vi "Load Plugins.vi"(8 "error in (no error)":errorcluster, 11 "Plugin Directories":path[](array[path])) -> (0 "error out":errorcluster, 3 "Plugin Array":T1[](array[typedef]))   [LabVIEW 2020, in "RxnRover.lvlib" / "Plugin Manager.lvlib"]
doc: "The core loader for plugins which initializes a Plugin Array, reads their configuration files and outputs a completed Plugin Array. This VI is currently called by Load Details and Filter Plugins. This VI calls several helper VIs starting with Read Plugins INI."
uses:
  Plugin Manager.lvlib
  Plugin Details.ctl
  Plugin Servers/Controller/Controller Type.ctl
  Plugin Types.ctl
  Config Error.ctl
  Plugin Servers/Controller/Generic Plugin.lvclass
  logging/logging.lvlib
panel:
  out "All Files in Dir":path[](array[path])
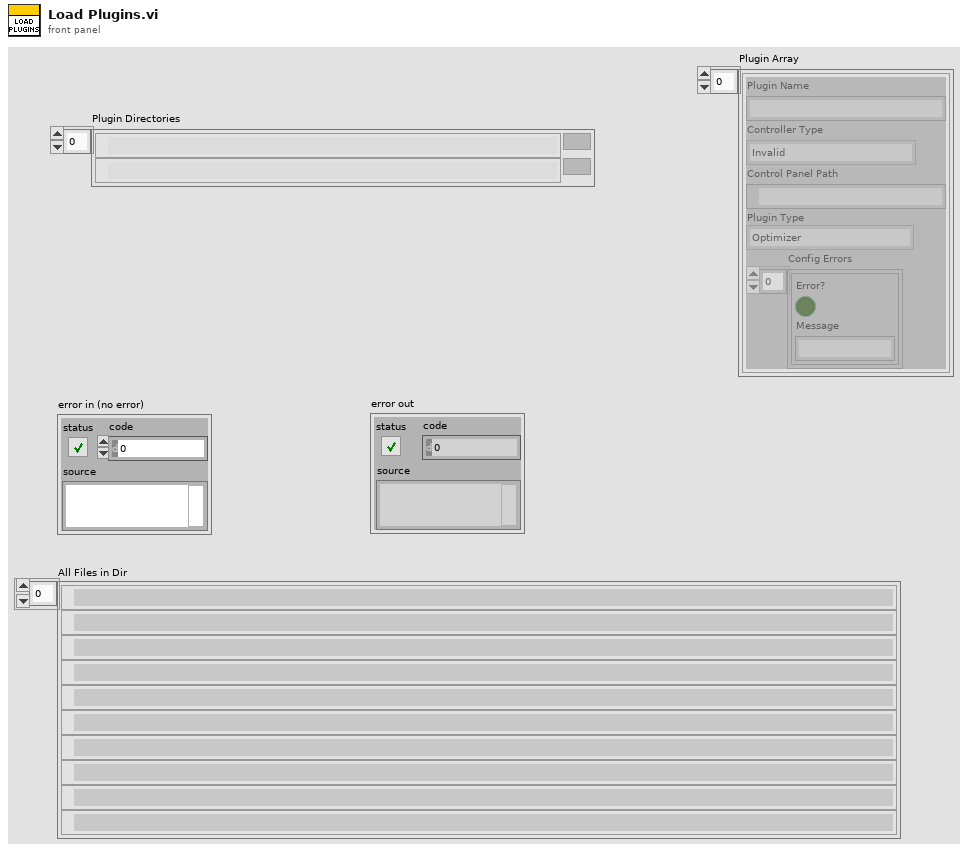
[diagram p1: front panel]
types:
  T1 = typedef "RxnRover.lvlib/Plugin Manager.lvlib/Plugin Details.ctl" = cluster{"Plugin Name":string, "Controller Type":T2, "Control Panel Path":path, "Plugin Type":T3, "Config Errors":T4[]}
  T2 = typedef "RxnRover.lvlib/Generic Plugin.lvclass/Controller Type.ctl" = enum16{"Invalid", "Temperature Controller", "Pump Controller", "Syringe Pump", "Generic Optimizer", "LC Parser", "Passive Hardware"}
  T3 = typedef "RxnRover.lvlib/Plugin Manager.lvlib/Plugin Types.ctl" = enum16{"Invalid", "Optimizer", "Analyzer", "Hardware"}
  T4 = typedef "RxnRover.lvlib/Plugin Manager.lvlib/Config Error.ctl" = cluster{"Error?":bool, "Message":string}
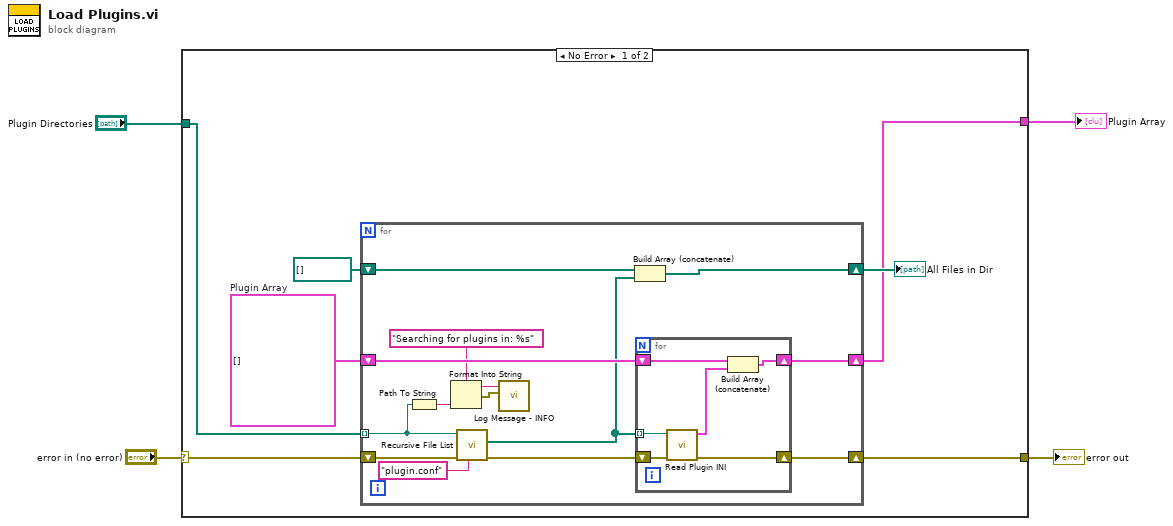
[diagram p0: block diagram]
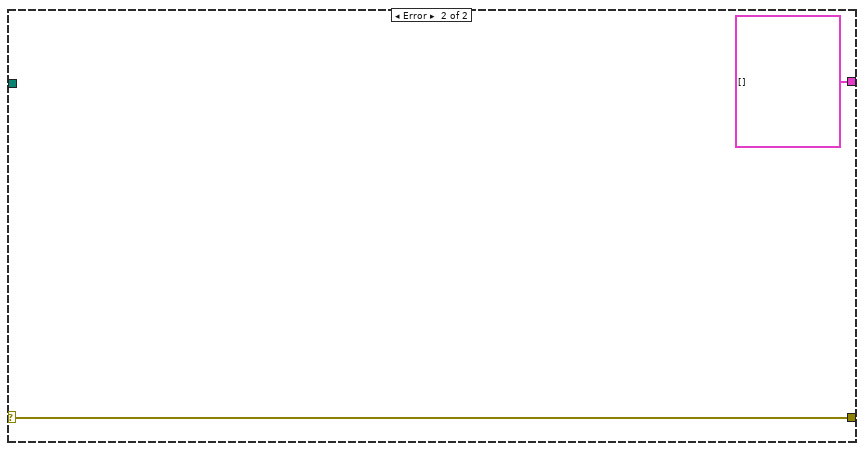
[diagram p2: hidden frame]
diagram:
  n1 = case shown="No Error" "error in (no error)" {
    selector: "error in (no error)" -> [w11 w33]
    tunnel: [w10 w33] -> w3
    tunnel: "Plugin Directories" -> [w8 _]
    tunnel: [w5 T1[] [] ("Plugin Array")] -> w2
    frame No Error {
      w9 = T1[] []  # Plugin Array
      n2 = for {
        shift-right: [w22] -> w10
        shift-left: w11 -> [w25]
        shift-right: [w20] -> w5
        shift-left: w9 -> [w21]
        tunnel: w8 -> [w13] mode=indexing
        shift-right: [w18] -> w6
        shift-left: path[] [] ("All Files in Dir") -> [w19]
        n3 = Path To String(path=w13) -> (string=w12:string)
        n4 = Format Into String(format string="Searching for plugins in: %s", w12) -> (resulting string=w15:string, error out=w16:errorcluster)  [unwired: 2 in]
        n5 = call <vilib>:"Recursive File List.vi"("pattern"="plugin.conf", "error in (no error)"=w25, "Folder Path"=w13) -> ("error out"=w23:errorcluster, "All Files in Dir"=w17:path[])  [unwired: 4 in, 3 out]
        n6 = call "Log Message - INFO.vi"("error in (no error)"=w16, "Message"=w15) -> ()  [unwired: 9 in, 1 out]
        n7 = Build Array (concatenate)(w19, w17) -> (w18:path[])
        n8 = for {
          shift-right: [w30] -> w22
          shift-left: w23 -> [w31]
          tunnel: w17 -> [w29] mode=indexing
          shift-right: [w27] -> w20
          shift-left: w21 -> [w28]
          n9 = call "Read Plugin INI.vi"("error in (no error)"=w31, "INI file"=w29) -> ("error out"=w30:errorcluster, "Plugin Details"=w26:T1)  [unwired: 8 in]
          n10 = Build Array (concatenate)(w28, w26) -> (w27:T1[])
        }
      }
      "All Files in Dir" <- w6
    }
    frame Error {
    }
  }
  "error out" <- w3
  "Plugin Array" <- w2
